vi "Num Convert Front Color.vi"(8 "error in (no error)":errorcluster, 9 "FTTColor":cluster{"Low":u32, "Middle":u32, "High":u32}, 10 "TargetRate":cluster{"Low":u32, "High":u32}, 11 "FTT Rate":string) -> (0 "error out":errorcluster, 3 "Middle":u32)   [LabVIEW 2014]
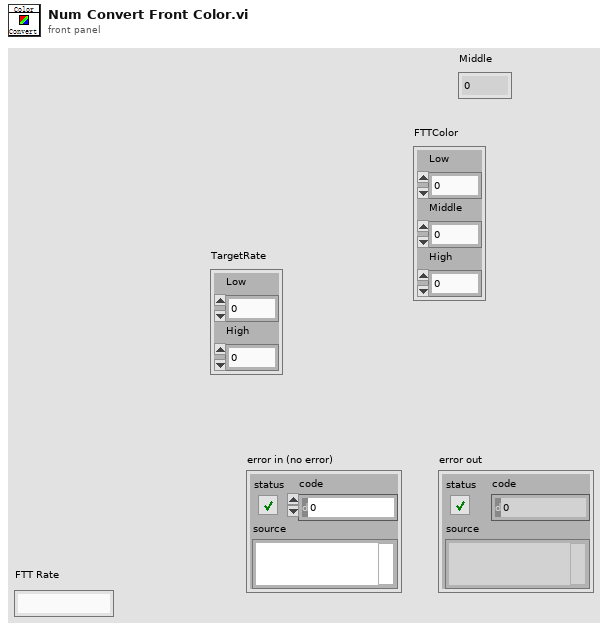
[diagram p1: front panel]
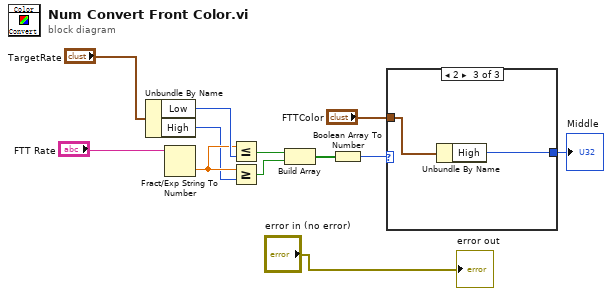
[diagram p0: block diagram]
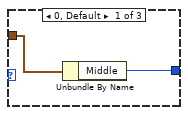
[diagram p2: hidden frame]
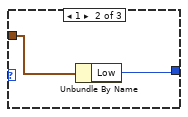
[diagram p3: hidden frame]
diagram:
  n1 = Unbundle By Name("TargetRate") -> ("Low"=w10:u32, "High"=w8:u32)
  n2 = Fract/Exp String To Number(string="FTT Rate") -> (number=w9:dbl)  [unwired: 3 in, 1 out]
  n3 = Less Or Equal?(x=w9, y=w10) -> (x <= y?=w7:bool)
  n4 = Greater Or Equal?(x=w9, y=w8) -> (x >= y?=w6:bool)
  n5 = Build Array(w7, w6) -> (w5:bool[])
  n6 = Boolean Array To Number(Boolean array=w5) -> (number=w4:u32)
  n7 = case shown="2" w4 {
    tunnel: "FTTColor" -> [w14 w16 w18]
    tunnel: [w13 w15 w17] -> w2
    frame 0, Default {
      n8 = Unbundle By Name(w14) -> ("Middle"=w13:u32)
    }
    frame 1 {
      n9 = Unbundle By Name(w16) -> ("Low"=w15:u32)
    }
    frame 2 {
      n10 = Unbundle By Name(w18) -> ("High"=w17:u32)
    }
  }
  "Middle" <- w2
  "error out" <- "error in (no error)"
